vi "Read Frame.vi"(8 "error in (no error)":errorcluster caption="entrée d'erreur (pas d'erreur)", 11 "Class Camera IV3-500CA (Default) en Entrée":refnum<class "Class Camera IV3-500CA.lvclass">) -> (0 "error out":errorcluster caption="sortie d'erreur", 3 "Class Camera IV3-500CA (Default) en Sortie":refnum<class "Class Camera IV3-500CA.lvclass">)   [LabVIEW 2020, in "Library Instrument & Equipement.lvlib" / "Library Camera.lvlib" / "Class Camera IV3-500CA.lvclass"]
uses:
  Class Camera IV3-500CA.lvclass
  C:/Users/ngarcin/OneDrive - Altyor/Standard TB/Class/Camera/Class Camera Pattern Matching (Default)/Class Pattern Matching (Default).lvclass
  Class Camera IV3-500CA.lvclass/Class Camera IV3-500CA.ctl
  Commun VI/Library Commun.lvlib
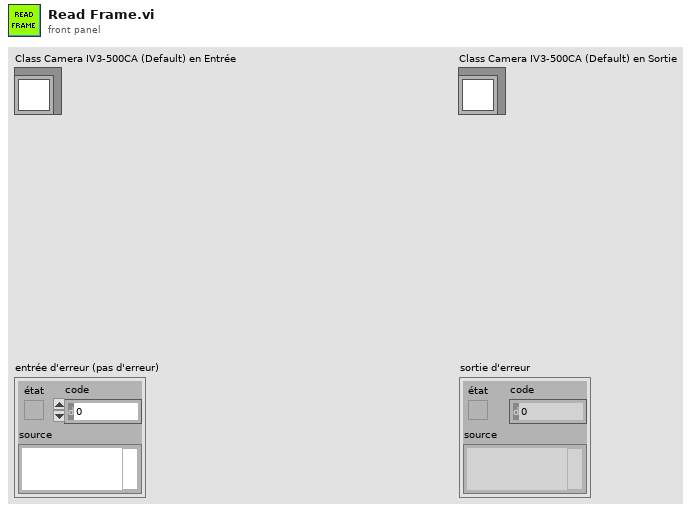
[diagram p1: front panel]
types:
  T1 = enum16{"Standard", "Buffered", "CRLF", "Immediate"}
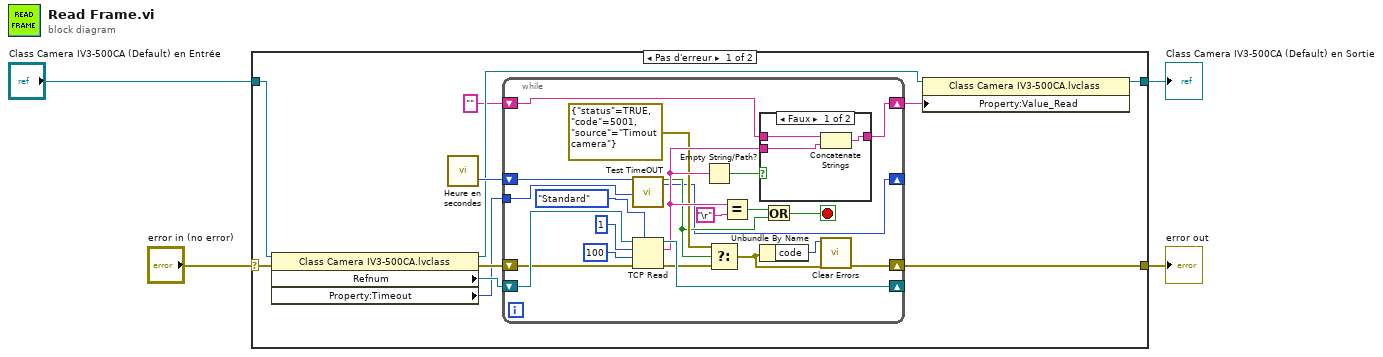
[diagram p0: block diagram]
diagram:
  n1 = case shown="Pas d'erreur" "error in (no error)" {
    selector: "error in (no error)" -> [w10 w43]
    tunnel: [w13 w43] -> w3
    tunnel: [w8 w42] -> w1
    tunnel: "Class Camera IV3-500CA (Default) en Entrée" -> [w15 w42]
    frame No Error {
      n2 = property class="Class Camera IV3-500CA.lvclass"(reference=w15, error in=w10) -> (reference out=w12:refnum<class "Class Camera IV3-500CA.lvclass">, error out=w9:errorcluster, "Refnum"=w11:refnum<k5>, "Property:Timeout"=w6:u16)
      n3 = call "Heure en secondes.vi"() -> ("Heure en milisecondes"=w14:u32)  [unwired: 2 in, 1 out]
      n4 = while {
        shift-right: [w37] -> _
        shift-left: w11 -> [w36]
        shift-right: [w29] -> w13
        shift-left: w9 -> [w35]
        shift-right: [w30] -> w7
        shift-left: "" -> [w31]
        shift-right: [w18] -> _
        shift-left: w14 -> [w20]
        tunnel: w6 -> [w16]
        stop <- w24 stop-if-true
        n5 = call "Test TimeOUT.vi"("OLD Time"=w20, "TimeOut ms"=w16) -> ("Timeout ?"=w19:bool, "NEW Time"=w18:u32)  [unwired: 13 in, 3 out]
        n6 = TCP Read(connection ID=w36, bytes to read=1, error in (no error)=w35, 7:T1."Standard" ("mode (standard)"), 9:100 ("timeout ms (25000)")) -> (connection ID out=w37:refnum<k5>, data out=w27:string, error out=w23:errorcluster)
        n7 = Empty String/Path?(string/path=w27) -> (empty?=w26:bool)
        n8 = Select(t=errorcluster {"status"=TRUE, "code"=5001, "source"="Timout camera"} ("cas vrai"), s=w19, f=w23) -> (s? t:f=w22:errorcluster)
        n9 = Equal?(x=w27, y="\r") -> (x = y?=w25:bool)
        n10 = case shown="Faux" w26 {
          tunnel: w31 -> [w40 w41]
          tunnel: [w39 w41] -> w30
          tunnel: w27 -> [w38 _]
          frame False {
            n11 = Concatenate Strings(w40, w38) -> (w39:string)
          }
          frame True {
          }
        }
        n12 = Unbundle By Name(w22) -> ("code"=w17:i32)
        n13 = Or(x=w25, y=w19) -> (x .or. y?=w24:bool)
        n14 = call <vilib>:"Clear Errors.vi"("error in (no error)"=w22, "specific error code to clear (0: all)"=w17) -> ("error out"=w29:errorcluster)  [unwired: 4 in, 1 out]
      }
      n15 = property class="Class Camera IV3-500CA.lvclass"(reference=w12, "Property:Value_Read"=w7) -> (reference out=w8:refnum<class "Class Camera IV3-500CA.lvclass">)  [unwired: 1 in, 1 out]
    }
    frame Error {
    }
  }
  "error out" <- w3
  "Class Camera IV3-500CA (Default) en Sortie" <- w1
